vi "Unflatten Boolean.vi"(11 "Tag value":string) -> (3 "Boolean":bool)   [LabVIEW 2020, in "NI_VIAn_XML Parsing.lvlib"]
uses:
  <vilib>/addons/analyzer/XML Parsing/NI_VIAn_XML Parsing.lvlib
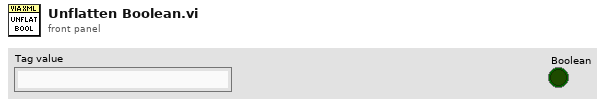
[diagram p1: front panel]
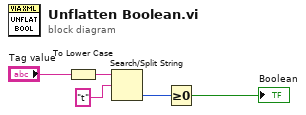
[diagram p0: block diagram]
diagram:
  n1 = To Lower Case(string="Tag value") -> (all lower case string=w2:string)
  n2 = Search/Split String(string=w2, search string/char (-)="t") -> (offset of match=w4:i32)  [unwired: 1 in, 2 out]
  n3 = Greater Or Equal To 0?(x=w4) -> (x >= 0?=→"Boolean":bool)
